vi "Open Application Reference.vi"() -> (0 "application reference":refnum<vi>)   [LabVIEW 2009]
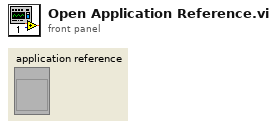
[diagram p1: front panel]
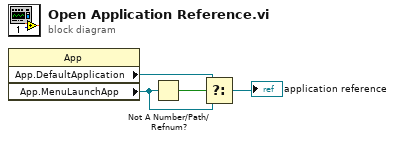
[diagram p0: block diagram]
diagram:
  n1 = property class="App"() -> ("App.DefaultApplication"=w1:refnum<vi>, "App.MenuLaunchApp"=w3:refnum<vi>)  [unwired: 2 in, 2 out]
  n2 = Not A Number/Path/Refnum?(number/path/refnum=w3) -> (NaN/Path/Refnum?=w4:bool)
  n3 = Select(t=w1, s=w4, f=w3) -> (s? t:f=→"application reference":refnum<vi>)
